vi "Find Unskipped Parent.vi"(10 "Start Index":i32, 11 "Graph In":T1[](array[typedef])) -> (1 "Index":i32, 2 "Found?":bool, 3 "Unskipped Parent":T1)   [LabVIEW 2020, in "Better Search.lvlib"]
uses:
  Better Search.lvlib
  Data Types/Type Reflection Item.ctl
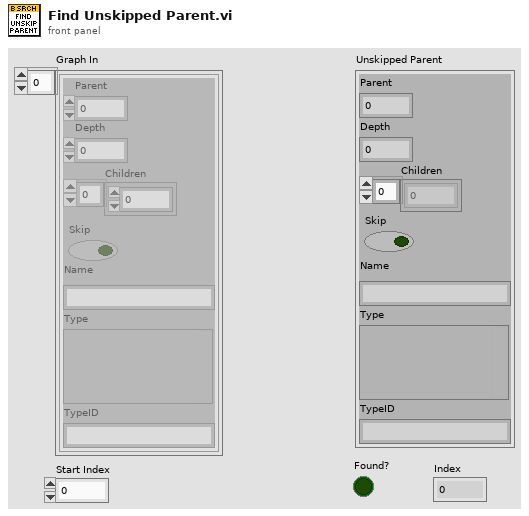
[diagram p1: front panel]
types:
  T1 = typedef "Better Search.lvlib/Type Reflection Item.ctl" = cluster{"Parent":i32, "Depth":i32, "Children":i32[], "Skip":bool, "Name":string, "Type":variant, "TypeID":string}
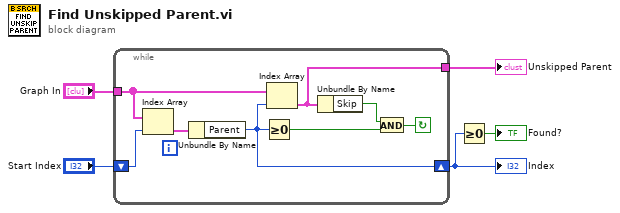
[diagram p0: block diagram]
diagram:
  n1 = while {
    shift-right: [w8] -> w2
    shift-left: "Start Index" -> [w10]
    tunnel: "Graph In" -> [w9]
    tunnel: [w6] -> w5
    stop <- w11 continue-if-true
    n2 = Index Array(array=w9, index=w10) -> (element=w13:T1)
    n3 = Unbundle By Name(w13) -> ("Parent"=w8:i32)
    n4 = Greater Or Equal To 0?(x=w8) -> (x >= 0?=w12:bool)
    n5 = Index Array(array=w9, index=w8) -> (element=w6:T1)
    n6 = Unbundle By Name(w6) -> ("Skip"=w7:bool)
    n7 = And(x=w7, y=w12) -> (x .and. y?=w11:bool)
  }
  "Unskipped Parent" <- w5
  "Index" <- w2
  n8 = Greater Or Equal To 0?(x=w2) -> (x >= 0?=→"Found?":bool)
